vi "New Auto.vi"   [LabVIEW 2013]
uses:
  <vilib>/Rock Robotics/WPI/RobotDrive/WPI_RobotDriveGetSetRefNum.vi
  <vilib>/Rock Robotics/WPI/RobotDrive/WPI_RobotDriveMecanumDrive_Cartesian.vi
types:
  T1 = typedef "WPI_RobotDriveDevRef.ctl" = cluster{"DevStatus":errorcluster, "Motors[]":T2[], "Square Inputs":bool, "Max Output":dbl, "Isochronous":bool}
  T2 = typedef "WPI_MotorControlDeviceRef.ctl" = cluster{"DeviceStatus":errorcluster, "Type":enum16{"PWM", "CAN"}, "PWM":cluster{"Digital Module":T3, "PWM Channel":T4, "DeadBand":T5}, "CAN":cluster{"Device Number":u8, "Control Mode":T6, "Semaphore":T7, "Max Vout":dbl}, "Invert":bool, "TransformRef":T8, "InvTransformRef":T8}
  T3 = typedef "FPGA_TypedefDigitalModule.ctl" = enum16{"Digital Module 1", "Digital Module 2"}
  T4 = typedef "FPGA_DIOPWMChannel.ctl" = enum8{"PWM 1", "PWM 2", "PWM 3", "PWM 4", "PWM 5", "PWM 6", "PWM 7", "PWM 8", "PWM 9", "PWM 10", "Invalid"}
  T5 = typedef "WPI_PWMDeadband.ctl" = cluster{"Name":string, "maxPositivePwm":i32, "minPositivePwm":i32, "centerPwm":i32, "maxNegativePwm":i32, "minNegativePwm":i32, "angularRange":u16}
  T6 = typedef "WPI_CANJaguar_ControlMode.ctl" = enum8{"Percent VBus", "Current", "Speed", "Position", "Voltage"}
  T7 = typedef "Semaphore RefNum" = refnum<k1>
  T8 = typedef "WPI_PWMTransform_ConPane.ctl" = refnum<vi>
  T9 = typedef "WPI_DigitalInputDevRef.ctl" = cluster{"DevStatus":errorcluster, "DIO Channel":T10, "Digital Module":T3}
  T10 = typedef "FPGA_DIOChannel.ctl" = enum8{"DIO 1", "DIO 2", "DIO 3", "DIO 4", "DIO 5", "DIO 6", "DIO 7", "DIO 8", "DIO 9", "DIO 10", "DIO 11", "DIO 12", "DIO 13", "DIO 14", "Invalid"}
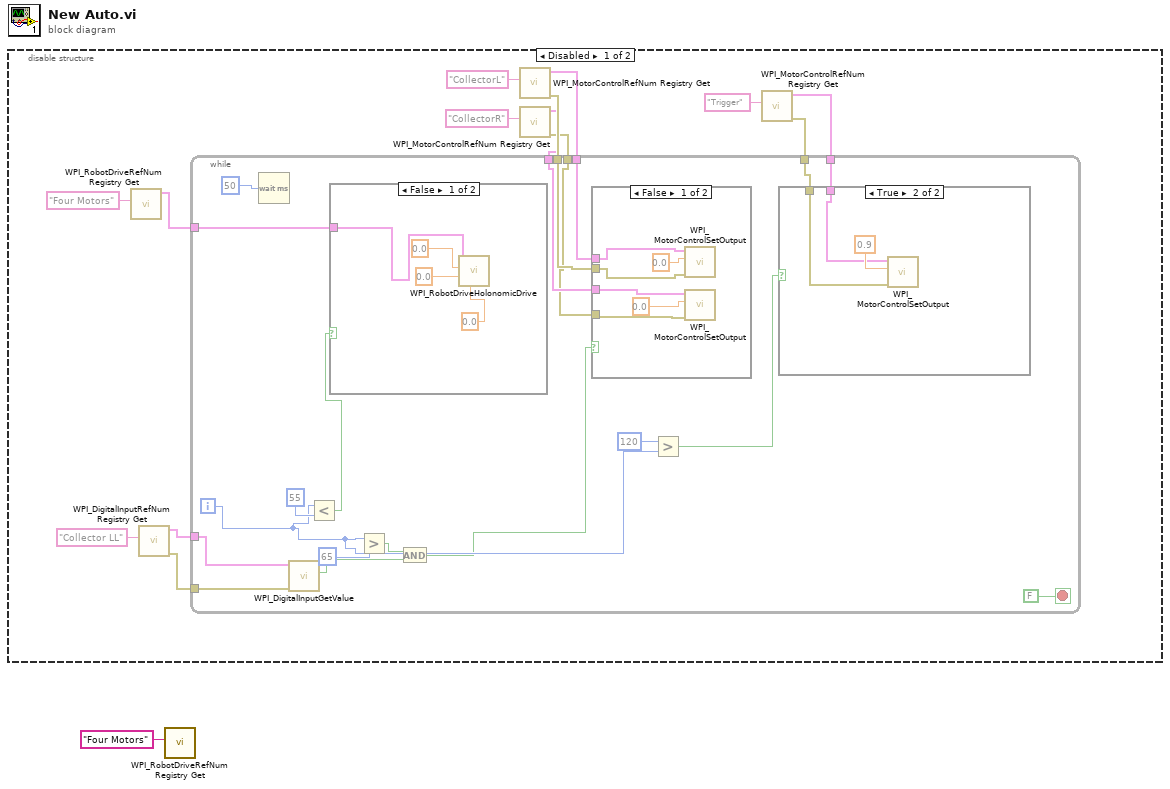
[diagram p0: block diagram]
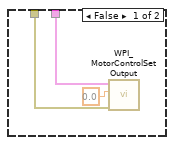
[diagram p2: hidden frame]
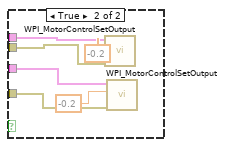
[diagram p3: hidden frame]
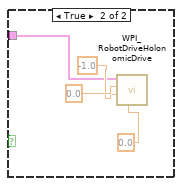
[diagram p4: hidden frame]
diagram:
  n1 = disable-structure shown="Disabled" {
    frame Disabled {
      n2 = call <vilib>:"WPI_RobotDriveRefNum Registry Get.vi"("refnum name"="Four Motors") -> ("RobotDriveDevRef"=w10:T1)  [unwired: 1 in, 9 out]
      n3 = call <vilib>:"WPI_DigitalInputRefNum Registry Get.vi"("refnum name"="Collector LL") -> ("error out"=w2:errorcluster, "DigitalInputDevRef"=w9:T9)  [unwired: 9 in]
      n4 = call <vilib>:"WPI_MotorControlRefNum Registry Get.vi"("refnum name"="CollectorL") -> ("error out"=w7:errorcluster, "MotorControlDevRef"=w8:T2)  [unwired: 9 in]
      n5 = call <vilib>:"WPI_MotorControlRefNum Registry Get.vi"("refnum name"="CollectorR") -> ("error out"=w5:errorcluster, "MotorControlDevRef"=w6:T2)  [unwired: 9 in]
      n6 = call <vilib>:"WPI_MotorControlRefNum Registry Get.vi"("refnum name"="Trigger") -> ("error out"=w3:errorcluster, "MotorControlDevRef"=w4:T2)  [unwired: 9 in]
      n7 = while {
        tunnel: w10 -> [w34]
        tunnel: w9 -> [w18]
        tunnel: w8 -> [w33]
        tunnel: w7 -> [w32]
        tunnel: w6 -> [w31]
        tunnel: w5 -> [w30]
        tunnel: w4 -> [w28]
        tunnel: w3 -> [w27]
        tunnel: w2 -> [w17]
        i -> [w21]
        stop <- FALSE stop-if-true
        n8 = Wait (ms)(milliseconds to wait=50) -> ()  [unwired: 1 out]
        n9 = call <vilib>:"WPI_DigitalInputGetValue.vi"("error in (no error)"=w17, "DigitalInputDevRef"=w18) -> ("Value"=w24:bool)  [unwired: 7 in, 2 out]
        n10 = Less?(x=w21, y=55 ("x")) -> (x < y?=w19:bool)
        n11 = case shown="False" w19 {
          tunnel: w34 -> [w54 w58]
          frame False {
            n12 = call-poly <vilib>:"WPI_RobotDriveHolonomicDrive.vi"("Rotation"=0.0, "Y"=0.0, "X"=0.0, "RobotDriveDevRef"=w54) -> ()  [unwired: 5 in, 3 out]
          }
          frame True {
            n13 = call-poly <vilib>:"WPI_RobotDriveHolonomicDrive.vi"("Rotation"=0.0, "Y"=-1.0, "X"=0.0, "RobotDriveDevRef"=w58) -> ()  [unwired: 5 in, 3 out]
          }
        }
        n14 = Greater?(x=w21, y=65 ("x")) -> (0:w25:bool)
        n15 = And(x=w25, y=w24) -> (x .and. y?=w20:bool)
        n16 = case shown="False" w20 {
          tunnel: w33 -> [w42 w51]
          tunnel: w32 -> [w43 w50]
          tunnel: w31 -> [w44 w49]
          tunnel: w30 -> [w45 w48]
          frame False {
            n17 = call <vilib>:"WPI_MotorControlSetOutput.vi"("error in (no error)"=w43, "Output"=0.0, "MotorControlDevRef"=w42) -> ()  [unwired: 6 in, 3 out]
            n18 = call <vilib>:"WPI_MotorControlSetOutput.vi"("error in (no error)"=w45, "Output"=0.0, "MotorControlDevRef"=w44) -> ()  [unwired: 6 in, 3 out]
          }
          frame True {
            n19 = call <vilib>:"WPI_MotorControlSetOutput.vi"("error in (no error)"=w50, "Output"=-0.2, "MotorControlDevRef"=w51) -> ()  [unwired: 6 in, 3 out]
            n20 = call <vilib>:"WPI_MotorControlSetOutput.vi"("error in (no error)"=w48, "Output"=-0.2, "MotorControlDevRef"=w49) -> ()  [unwired: 6 in, 3 out]
          }
        }
        n21 = Greater?(x=120, y=w21) -> (0:w26:bool)
        n22 = case shown="True" w26 {
          tunnel: w28 -> [w37 w39]
          tunnel: w27 -> [w36 w40]
          frame False {
            n23 = call <vilib>:"WPI_MotorControlSetOutput.vi"("error in (no error)"=w36, "Output"=0.0, "MotorControlDevRef"=w37) -> ()  [unwired: 6 in, 3 out]
          }
          frame True {
            n24 = call <vilib>:"WPI_MotorControlSetOutput.vi"("error in (no error)"=w40, "Output"=0.9, "MotorControlDevRef"=w39) -> ()  [unwired: 6 in, 3 out]
          }
        }
      }
    }
    frame Enabled {
    }
  }
  n25 = call <vilib>:"WPI_RobotDriveRefNum Registry Get.vi"("refnum name"="Four Motors") -> ()  [unwired: 1 in, 10 out]
